vi "Write Data and Memory Array.vi"(4 "Secondary / Imaginary (0.0)":dbl[](array[numeric]), 6 "Primary / Real (0.0)":dbl[](array[numeric]), 7 "Channel (1)":i32=1, 8 "error in (no error)":errorcluster, 9 "Correction (0: Formatted)":u16(ring) items=["Formatted", "Corrected"], 10 "Source (0: Data)":u16(ring) items=["Data", "Memory"], 11 "VISA resource name":refnum<visa-resource-name>) -> (0 "error out":errorcluster, 3 "VISA resource name out":refnum<visa-resource-name>)   [LabVIEW 2022 SP3, in "Agilent ENA Series.lvlib"]
doc: "Sets the formated or corrected data or memory array, for the active trace of selected channel."
uses:
  <instrlib>/Agilent ENA Series/Agilent ENA Series.lvlib
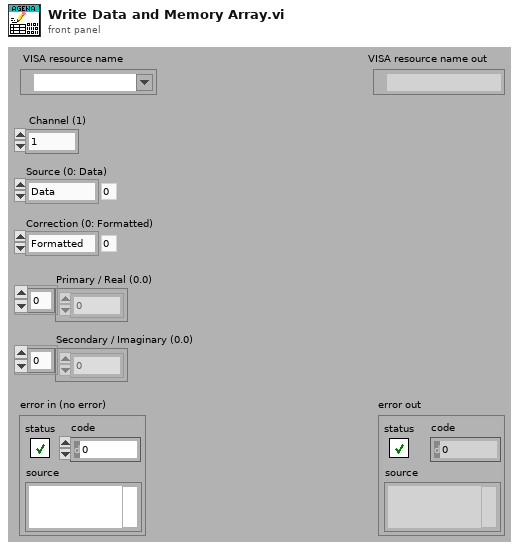
[diagram p1: front panel]
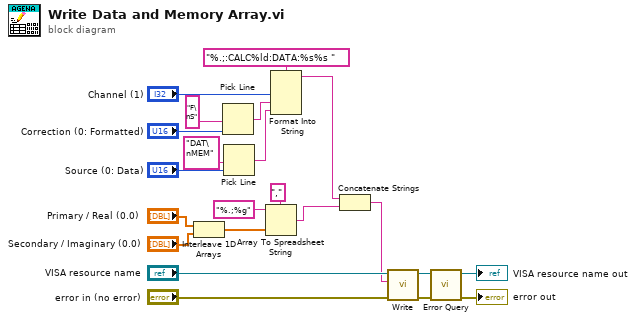
[diagram p0: block diagram]
diagram:
  n1 = Interleave 1D Arrays("Primary / Real (0.0)", "Secondary / Imaginary (0.0)") -> (w7:dbl[])
  n2 = Pick Line(multi-line string="F\nS", line index="Correction (0: Formatted)") -> (output string=w15:string)  [unwired: 1 in]
  n3 = Pick Line(multi-line string="DAT\nMEM", line index="Source (0: Data)") -> (output string=w12:string)  [unwired: 1 in]
  n4 = Array To Spreadsheet String(delimiter (Tab)=",", array=w7, 3:"%.;%g" ("format string")) -> (spreadsheet string=w6:string)
  n5 = Format Into String(format string="%.;:CALC%ld:DATA:%s%s ", "Channel (1)", w15, w12) -> (resulting string=w11:string)  [unwired: 2 in, 1 out]
  n6 = Concatenate Strings(w11, w6) -> (w5:string)
  n7 = call <instrlib>:"Write.vi"("error in (no error)"="error in (no error)", "String ()"=w5, "VISA resource name"="VISA resource name") -> ("error out"=w3:errorcluster, "VISA resource name out"=w4:refnum<visa-resource-name>)  [unwired: 6 in, 1 out]
  n8 = call <instrlib>:"Error Query.vi"("error in (no error)"=w3, "VISA resource name"=w4) -> ("error out"=→"error out":errorcluster, "VISA resource name out"=→"VISA resource name out":refnum<visa-resource-name>)  [unwired: 6 in, 2 out]
